vi "NotUse_54_UNDT_ReceiverStaticGainParam (SubVI).vi"(8 "error in":errorcluster, 10 "ReceiverStaticGainParam":T1(ring), 11 "String in":refnum<vi>) -> (0 "error out":errorcluster)   [LabVIEW 2017]
uses:
  Global_SNK3_HF.vi
  LV_Unicorn/LV_Unicorn.lvlib
panel:
  in  "Dbl":i32 min=0 max=40
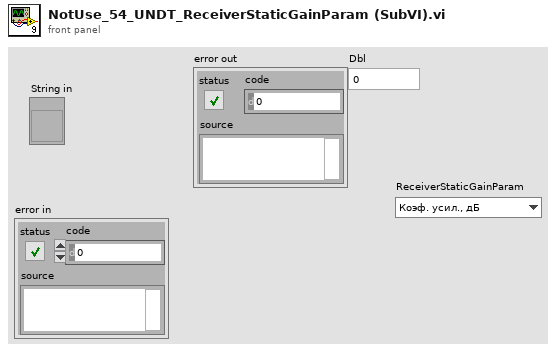
[diagram p1: front panel]
types:
  T1 = enum16{"Коэф. усил., дБ", "Вых. ЦАП (10 бит)", "Вых. ЦАП "}
  T2 = typedef "LV_Unicorn.lvlib/unicorn_Param.ctl" = cluster{"conParam":T3, "Param":T4}
  T3 = typedef "LV_Unicorn.lvlib/unicorn_conn.ctl" = cluster{"ReadIntParam":bool, "ReadDescrParam":bool, "ReadFloatParam":bool, "debug":bool, "ReadJSON":bool, "IP_address":string, "N_attempts":i32, "type_con":enum16{"Serial", "TCP"}, "MB_address":i32, "VISA":refnum<visa-resource-name>, "connection ID":refnum<k5>, "nameDevices":string, "timeout":i32, "port":u16, "type_version":string, "baud_rate":u32, "VersionControl":bool, "TCP_conn":bool, "WindowSize":i32}
  T4 = typedef "LV_Unicorn.lvlib/unicorn_JSON.ctl" = cluster{"NumParam":cluster{"NTelem":i32, "NInt":i32, "NFloat":i32, "NTable":i32}, "ParamInt":T5, "Telemetry":T6, "Table":T7, "ParamFloat":T8}
  T5 = typedef "LV_Unicorn.lvlib/unicorn_ParamInt.ctl" = cluster{"ID":string, "Num":i32, "Name":string, "Type":string, "Enum":string, "Desc":string, "Unit":string, "Access":string, "FormatStr":string, "Min":i32, "Max":i32}[]
  T6 = typedef "LV_Unicorn.lvlib/unicorn_Telemetry.ctl" = cluster{"ID":string, "Num":i32, "Name":string, "Desc":string, "Unit":string, "FormatStr":string, "Min":i32, "Max":i32}[]
  T7 = typedef "LV_Unicorn.lvlib/unicorn_Table.ctl" = cluster{"Num":i32, "Access":string, "ColumnCount":i32, "NeedParamPrepare":bool, "Columns":cluster{"Column":i32, "Desc":string, "Name":string}[], "DataType":string, "FormatStr":string, "ID":string, "Name":string, "RowCount":i32, "Rows":cluster{"Desc":string, "ID":string, "Max":i32, "Min":i32, "Name":string, "Row":i32, "Unit":string}[], "Type":string}[]
  T8 = typedef "LV_Unicorn.lvlib/unicorn_ParamFloat.ctl" = cluster{"ID":string, "Num":i32, "Name":string, "Type":string, "Enum":string, "Desc":string, "Unit":string, "Access":string, "FormatStr":string, "Min":sgl, "Max":sgl}[]
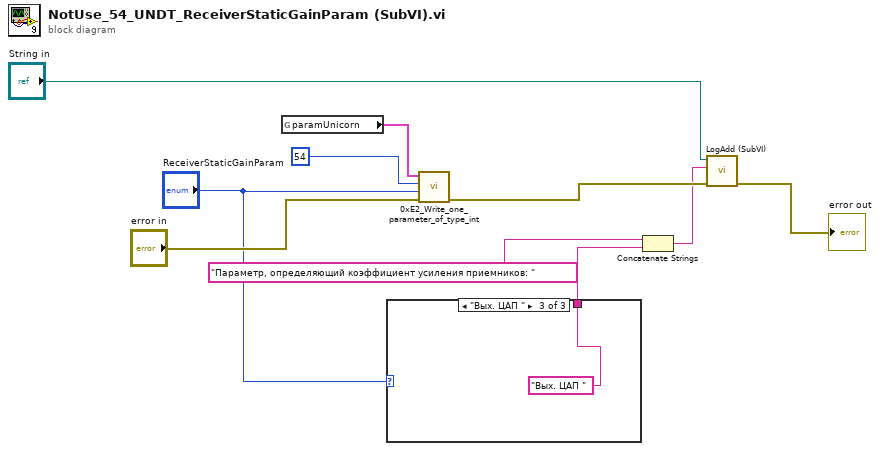
[diagram p0: block diagram]
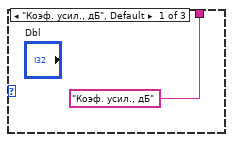
[diagram p2: hidden frame]
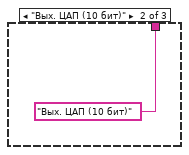
[diagram p3: hidden frame]
diagram:
  n1 = global read "Global_SNK3_HF.vi" "paramUnicorn"() -> (w8:T2)
  n2 = case shown="\"Вых. ЦАП \"" "ReceiverStaticGainParam" {
    tunnel: ["Коэф. усил., дБ" ("string") "Вых. ЦАП (10 бит)" ("string") "Вых. ЦАП " ("string")] -> w2
    frame "Коэф. усил., дБ", Default {
    }
    frame "Вых. ЦАП (10 бит)" {
    }
    frame "Вых. ЦАП " {
    }
  }
  n3 = call "0xE2_Write_one_parameter_of_type_int.vi"("error in"="error in", "ParamIn"="ReceiverStaticGainParam", "NumParamIn"=54 ("Номер параметра"), "paramUnicorn 2"=w8) -> ("error out"=w10:errorcluster)  [unwired: 4 in, 3 out]
  n4 = Concatenate Strings("Параметр, определяющий коэффициент усиления приемников: " ("string"), w2) -> (w4:string)
  n5 = call "LogAdd (SubVI).vi"("error in"=w10, "string"=w4, "Log"="String in") -> ("error out"=→"error out":errorcluster)  [unwired: 8 in]
